vi "CMD_Loop.vi"() -> ()   [LabVIEW 2023, in "2023-Auto_CMD.lvlib"]
uses:
  2023-Auto_CMD.lvlib
  Cluster_CMD_CMD_Data.ctl
  Shared Code/TypeDefs/ENUM_AutoSelect.ctl
  ENUM_CMD_State.ctl
  ENUM_CMD_Action.ctl
  Shared Code/TypeDefs/Cluster_AutoSequence.ctl
  Shared Code/TypeDefs/Cluster_Auto Sequence Data.ctl
  Shared Code/TypeDefs/Cluster_Auto Sequence Settings.ctl
  ENUM_Drive Mode Select.ctl
  Shared Code/TypeDefs/Dial_Compase heading unit circle CCW positive.ctl
  Shared Code/TypeDefs/Cluster_Module Velocity-Direction-Rotations.ctl
  Shared Code/TypeDefs/Level_Velocity plus-minus 1.ctl
  SwerveDrive/Cluster_CMD_ACT_Data.ctl
  Shared Code/TypeDefs/ENUM_CMD_Mode Select.ctl
  Shared Code/TypeDefs/Cluster_CMD_Direction Data.ctl
  Shared Code/TypeDefs/Cluster_X-Y.ctl
  Shooter/Cluster_CMD_ACT_Data.ctl
  Shooter/ENUM_Shooter_Mode.ctl
  <vilib>/Rock Robotics/WPI/DriverStation/WPI_DriverStationRobotMode2.ctl
  Shared Code/TypeDefs/Cluster_Config_AutoData.ctl
  Pivot FX/Cluster_CMD_ACT_Data.ctl
  Pivot FX/ENUM_CMD_Mode Select.ctl
  Shared Code/TypeDefs/ENUM_Pivot Arm Position Select.ctl
  fdd46993-b9fc-440f-aafb-7ab1a8c35176.vi
  133b30be-2fcb-456e-b4b0-07f770c500ae.vi
  1ba0cf27-86ce-4142-8b65-bcb405614ff3.vi
  09229b25-3731-4416-b61c-801146eec302.vi
  c7d6c6c0-b27b-4b8b-8552-511dbe9cf3c3.vi
  dfaa9063-9cc7-40d1-a81d-c10c38088b54.vi
  fdd46993-b9fc-440f-aafb-7ab1a8c35176.vi/958b2683-dd4b-41b7-8ed1-41c95f63cef0.vi
  fdd46993-b9fc-440f-aafb-7ab1a8c35176.vi/95f5fa9b-6175-4b34-88ee-cece92c38279.vi
  133b30be-2fcb-456e-b4b0-07f770c500ae.vi/958b2683-dd4b-41b7-8ed1-41c95f63cef0.vi
  133b30be-2fcb-456e-b4b0-07f770c500ae.vi/95f5fa9b-6175-4b34-88ee-cece92c38279.vi
  09229b25-3731-4416-b61c-801146eec302.vi/958b2683-dd4b-41b7-8ed1-41c95f63cef0.vi
  09229b25-3731-4416-b61c-801146eec302.vi/95f5fa9b-6175-4b34-88ee-cece92c38279.vi
  c7d6c6c0-b27b-4b8b-8552-511dbe9cf3c3.vi/958b2683-dd4b-41b7-8ed1-41c95f63cef0.vi
  c7d6c6c0-b27b-4b8b-8552-511dbe9cf3c3.vi/95f5fa9b-6175-4b34-88ee-cece92c38279.vi
  <vilib>/Utility/error.llb/Trim Whitespace.vi
  fdd46993-b9fc-440f-aafb-7ab1a8c35176.vi/95f5fa9b-6175-4b34-88ee-cece92c38279.vi/1c6bd52c-bbca-4d4a-a290-93ea2703fded.vi
  fdd46993-b9fc-440f-aafb-7ab1a8c35176.vi/95f5fa9b-6175-4b34-88ee-cece92c38279.vi/47c2b0d5-b5fa-444e-9535-611565d375db.vi
  133b30be-2fcb-456e-b4b0-07f770c500ae.vi/95f5fa9b-6175-4b34-88ee-cece92c38279.vi/1c6bd52c-bbca-4d4a-a290-93ea2703fded.vi
  133b30be-2fcb-456e-b4b0-07f770c500ae.vi/95f5fa9b-6175-4b34-88ee-cece92c38279.vi/47c2b0d5-b5fa-444e-9535-611565d375db.vi
  09229b25-3731-4416-b61c-801146eec302.vi/95f5fa9b-6175-4b34-88ee-cece92c38279.vi/1c6bd52c-bbca-4d4a-a290-93ea2703fded.vi
  09229b25-3731-4416-b61c-801146eec302.vi/95f5fa9b-6175-4b34-88ee-cece92c38279.vi/47c2b0d5-b5fa-444e-9535-611565d375db.vi
  c7d6c6c0-b27b-4b8b-8552-511dbe9cf3c3.vi/95f5fa9b-6175-4b34-88ee-cece92c38279.vi/1c6bd52c-bbca-4d4a-a290-93ea2703fded.vi
  c7d6c6c0-b27b-4b8b-8552-511dbe9cf3c3.vi/95f5fa9b-6175-4b34-88ee-cece92c38279.vi/47c2b0d5-b5fa-444e-9535-611565d375db.vi
  <vilib>/Utility/error.llb/Trim Whitespace One-Sided.vi
  Robot Global Data.vi
  RoboRIO Utilities/Global_STOP.vi
  <vilib>/Utility/Data Type/Get Type Information.vi
  Shared Code/Utility/RWA/RWA/File/RWA_PC FIle Read String.vi
  Shared Code/Utility/RWA/RWA/Read Write Anything/RWA_File String.vi
  Shared Code/Utility/RWA/RWA/File/RWA_PC File Write String.vi
  Global_CMD_CMD_Data In.vi
  Shooter/Global_ACT_Data Out.vi
  SwerveDrive/Global_ACT_Data Out.vi
  Pivot FX/Global_ACT_Data Out.vi
  Pivot FX/Global_CMD_ACT_Data In.vi
  Shooter/Global_CMD_ACT_Data In.vi
  SwerveDrive/Global_CMD_ACT_Data In.vi
  Global_CMD_Data Out.vi
  <vilib>/Comparison/Equal/Equal Functor/Equal Functor.lvclass
  SwerveDrive/SwerveDrive_ACT_ts.lvlib
  Shooter/Shooter_ACT.lvlib
  Pivot FX/Pivot FX_ACT.lvlib
panel:
  out "Encoder .Position":i32
  out "Pivot at Position":bool
  out "Sequence Data":T1={"State"=enum."Starting", "Max Wait Time (S)"=0.0, "CMDs"={"Drive Mode"=enum."Wait", "Auto Angle"=0.0, "Traverse"={"Velocity"=0.0, "Angle"=0.0, "Rotations Count"=0.0}, "Shooter Speed"=0.0}, "Color Box"=16448250} {"CMDs"."Traverse"."Angle" scale format="%.3f"; "CMDs"."Traverse"."Velocity" scale=-1.0..1.0 scale format="%.1f"; "CMDs"."Auto Angle" scale format="%.3f"}
  out "CMD_Shooter":T8
  out "CMD_SwerveDrive":T10 {"Auto Angle" scale format="%.3f"; "Direction"."Rotate(Yaw) CCW 1 CW -1" scale=1.0..-1.0; "Direction"."Traverse"."Angle" scale format="%.3f"; "Direction"."Traverse"."Velocity" scale=-1.0..1.0 scale format="%.1f"}
  in  "AutoData.Sequences":T14[](array[typedef])=[{"Name"=enum."Unknown", "List"=[{"State"=enum."Driving to Position", "Max Wait Time (S)"=2.0, "CMDs"={"Drive Mode"=enum."Wait", "Auto Angle"=0.0, "Traverse"={"Velocity"=0.3, "Angle"=0.0, "Rotations Count"=0.0}, "Shooter Speed"=0.0}, "Color Box"=8404992}]}] {"List"."CMDs"."Traverse"."Angle" scale format="%.3f"; "List"."CMDs"."Traverse"."Velocity" scale=-1.0..1.0 scale format="%.1f"; "List"."CMDs"."Auto Angle" scale format="%.3f"}
  out "Remaing Match Time":sgl
  out "Step Index 2":i32
  out "CMD Input.Auto Select":T15=enum."Shoot and Drive Center"
  out "Found":bool
  out "Error Out":errorcluster
  out "Message Out":string
  in  "Read Saved Config":bool
  in  "Update Config":bool
  out "Action":T16
  out "State":T2
  out "Step Index":i32
  out "CMD_CMD_2022-Auto_Data":T17={"Auto Select"=enum."Shoot and Drive SpeakerLeft"}
  in  "Reset Sequence":bool
  in  "Reset All":bool
  in  "Set Manual":bool
  out "Input Data":T17={"Auto Select"=enum."Shoot and Drive SpeakerLeft"}
  out "Cycle Time (S)":dbl format="%.3g"
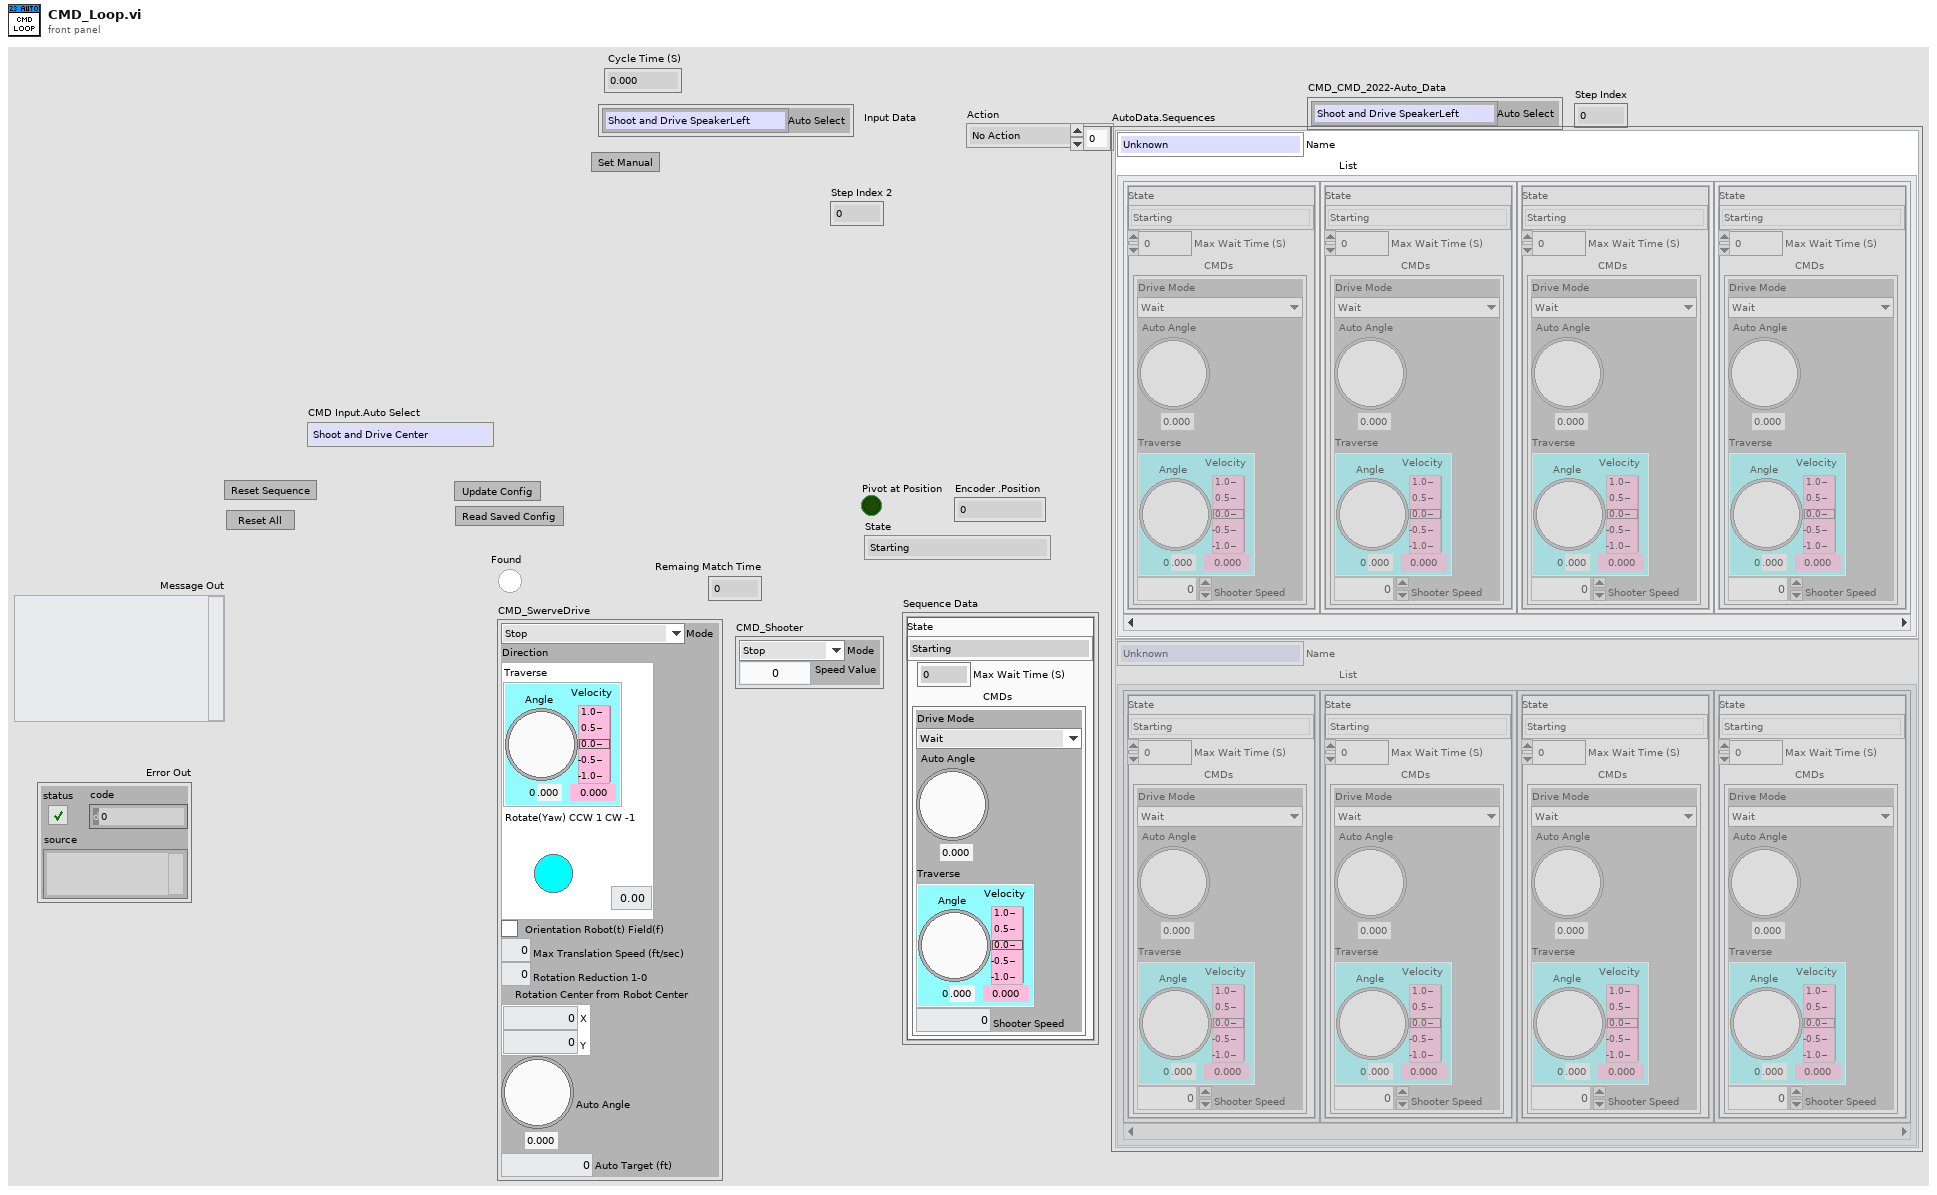
[diagram p1: front panel]
types:
  T1 = typedef "Cluster_Auto Sequence Data.ctl" = cluster{"State":T2, "Max Wait Time (S)":dbl, "CMDs":T3, "Color Box":u32}
  T2 = typedef "2023-Auto_CMD.lvlib/ENUM_CMD_State.ctl" = enum16{"Starting", "Idling", "Selecting Sequence", "Selecting Next Step", "Driving to Position", "Stopping", "Waiting", "Shutting Down", "Configuring", "Shooting", "Waiting for Pivot"}
  T3 = typedef "Cluster_Auto Sequence Settings.ctl" = cluster{"Drive Mode":T4, "Auto Angle":T5, "Traverse":T6, "Shooter Speed":dbl}
  T4 = typedef "2023-Auto_CMD.lvlib/ENUM_Drive Mode Select.ctl" = enum16{"Wait", "Timed Direction Drive", "Rotate to Angle", "Stop", "Auto Shoot"}
  T5 = typedef "Dial_Compase heading unit circle CCW positive.ctl" = dbl
  T6 = typedef "Cluster_Module Velocity-Direction-Rotations.ctl" = cluster{"Velocity":T7, "Angle":T5, "Rotations Count":dbl}
  T7 = typedef "Level_Velocity plus-minus 1.ctl" = dbl
  T8 = typedef "Shooter_ACT.lvlib/Cluster_CMD_ACT_Data.ctl" = cluster{"Mode":T9, "Speed Value":dbl}
  T9 = typedef "Shooter_ACT.lvlib/ENUM_Shooter_Mode.ctl" = enum16{"Stop", "Speed Percent", "Speed RPM", "AutoShoot"}
  T10 = typedef "SwerveDrive_ACT_ts.lvlib/Cluster_CMD_ACT_Data.ctl" = cluster{"Mode":T11, "Direction":T12, "Orientation Robot(t) Field(f)":bool, "Max Translation Speed (ft/sec)":dbl, "Rotation Reduction 1-0":dbl, "Rotation Center from Robot Center":T13, "Auto Angle":T5, "Auto Target (ft)":dbl}
  T11 = typedef "ENUM_CMD_Mode Select.ctl" = enum16{"Stop", "Translate Cmd Rotate Cmd", "Translate Cmd Rotate Auto"}
  T12 = typedef "Cluster_CMD_Direction Data.ctl" = cluster{"Traverse":T6, "Rotate(Yaw) CCW 1 CW -1":dbl}
  T13 = typedef "Cluster_X-Y.ctl" = cluster{"X":dbl, "Y":dbl}
  T14 = typedef "Cluster_AutoSequence.ctl" = cluster{"Name":T15, "List":T1[]}
  T15 = typedef "ENUM_AutoSelect.ctl" = enum16{"Unknown", "Shoot and Drive Center", "Shoot and Drive SpeakerLeft", "Shoot and Drive SpeakerRight"}
  T16 = typedef "2023-Auto_CMD.lvlib/ENUM_CMD_Action.ctl" = enum16{"No Action", "Reset Time", "Reset All", "Set System Cmds", "Reset Sequence", "Config File Read", "Config File Wirte", "Config from FP"}
  T17 = typedef "2023-Auto_CMD.lvlib/Cluster_CMD_CMD_Data.ctl" = cluster{"Auto Select":T15}
  T18 = typedef "Cluster_Config_AutoData.ctl" = cluster{"AutoData Ver":u64, "Sequences":T14[]}
  T19 = typedef "WPI_DriverStationRobotMode2.ctl" = enum16{"Autonomous Disabled", "Autonomous Enabled", "Teleop Disabled", "Teleop Enabled", "Disconnected", "Finish", "Test Disabled", "Test Enabled", "Emergency Stopped"}
  T20 = cluster{"State":T2, "Previous State":T2, "Current Time":timestamp, "Previous Time":timestamp, "Start Time":timestamp, "Target Time (ms)":u32, "Cycle Time(S)":dbl, "CMD Input":T17, "Sequence Array":T1[], "Step Data":T3, "Step Index":i32, "Robot Mode":T19, "Prev Robot Mode":T19, "Auto Select ":T15, "Team Files Folder":path, "AutoData":T18, "Update Display":bool, "Data Read":bool, "Remaing Match Time":sgl, "CMD_SwerveDrive":T10, "CMD_Shooter":T8, "AutoShootComplete":bool, "AutoAngleComplete":bool, "Pivot Out of the way":bool}
  T21 = typedef "Pivot FX_ACT.lvlib/Cluster_CMD_ACT_Data.ctl" = cluster{"Mode":T22, "Percent":dbl, "Target Position":dbl, "Position Select":T23}
  T22 = typedef "Pivot FX_ACT.lvlib/ENUM_CMD_Mode Select.ctl" = enum16{"STOP", "PercentOut", "Positon Value", "Position Select"}
  T23 = typedef "ENUM_Pivot Arm Position Select.ctl" = enum16{"Full Back", "Full Forward", "Amp Score", "Pivot Arm Load", "Vertical", "Trap Score"}
  T24 = typedef "SwerveDrive_ACT_ts.lvlib/Cluster_System Output Data.ctl" = cluster{"At Angle":bool}
  T25 = typedef "Pivot FX_ACT.lvlib/Cluster_HW Output Values.ctl" = cluster{"CLosed Loop":T26, "Current":T27, "Limit Switches":T28, "Voltage Values":T29, "Encoder ":T30}
  T26 = typedef "Cluster_FX CloseLoop Values.ctl" = cluster{"Target":dbl, "Error":i32, "Error D":dbl, "I Accum":dbl}
  T27 = typedef "Cluster_FX Current Values.ctl" = cluster{"Supply":dbl, "Stator":dbl}
  T28 = typedef "Cluster_FX Limit Switchs.ctl" = cluster{"FWD Closed":bool, "REV Closed":bool}
  T29 = typedef "Cluster_FX Voltage Values.ctl" = cluster{"Percent Output":dbl, "Output Voltage":dbl, "Bus Voltage":dbl}
  T30 = typedef "Cluster_FX Sensor Values.ctl" = cluster{"Position":i32, "Velocity":i32}
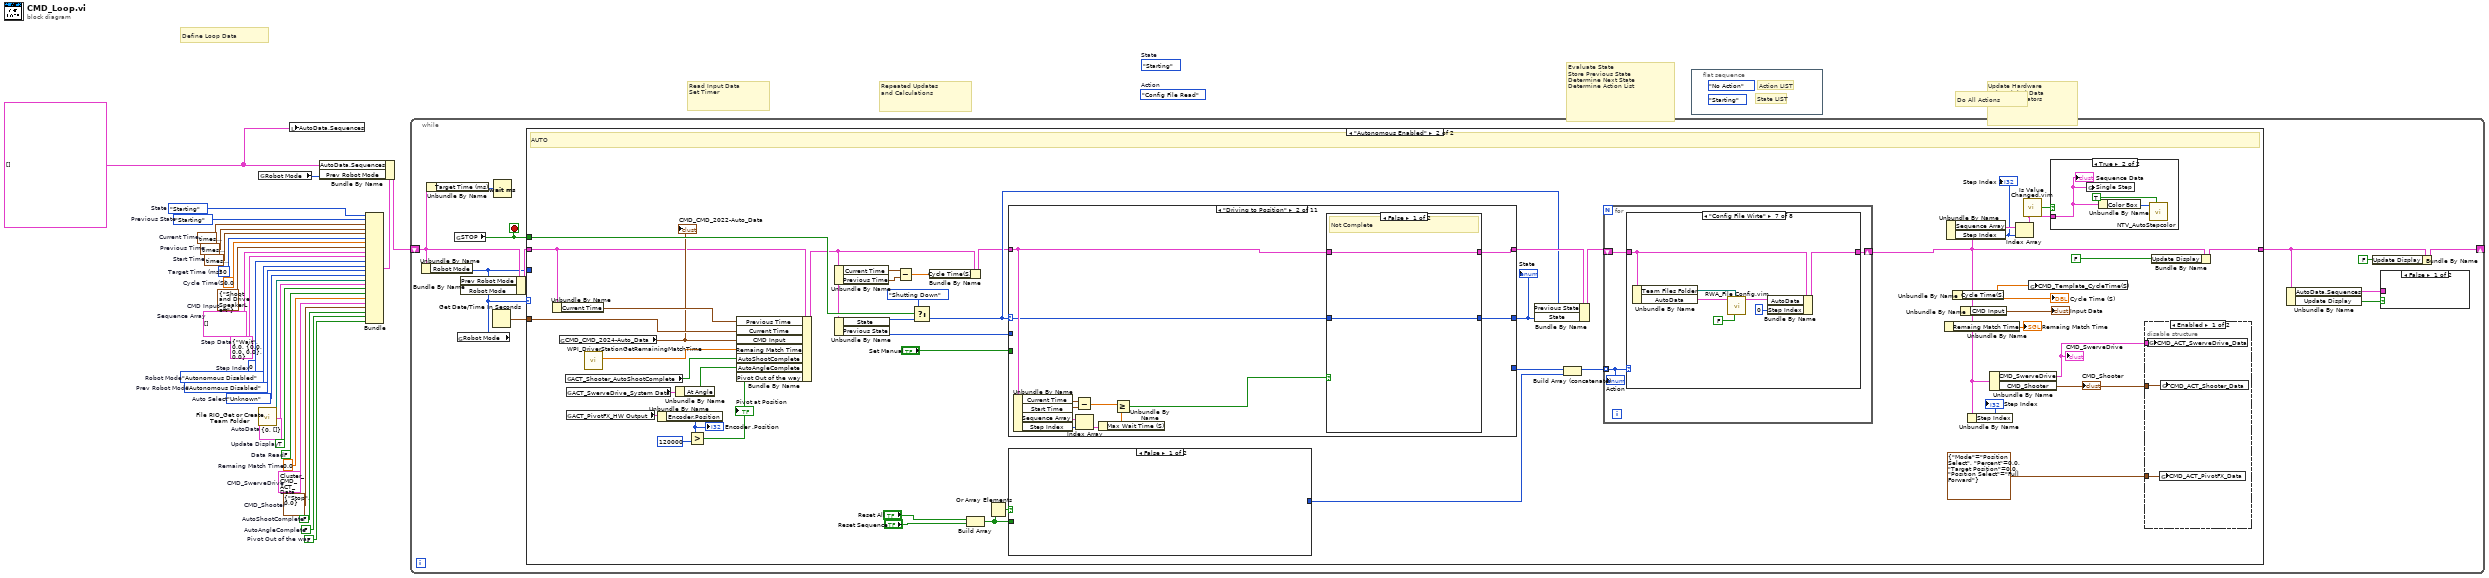
[diagram p0: block diagram]
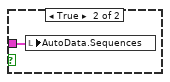
[diagram p2: hidden frame]
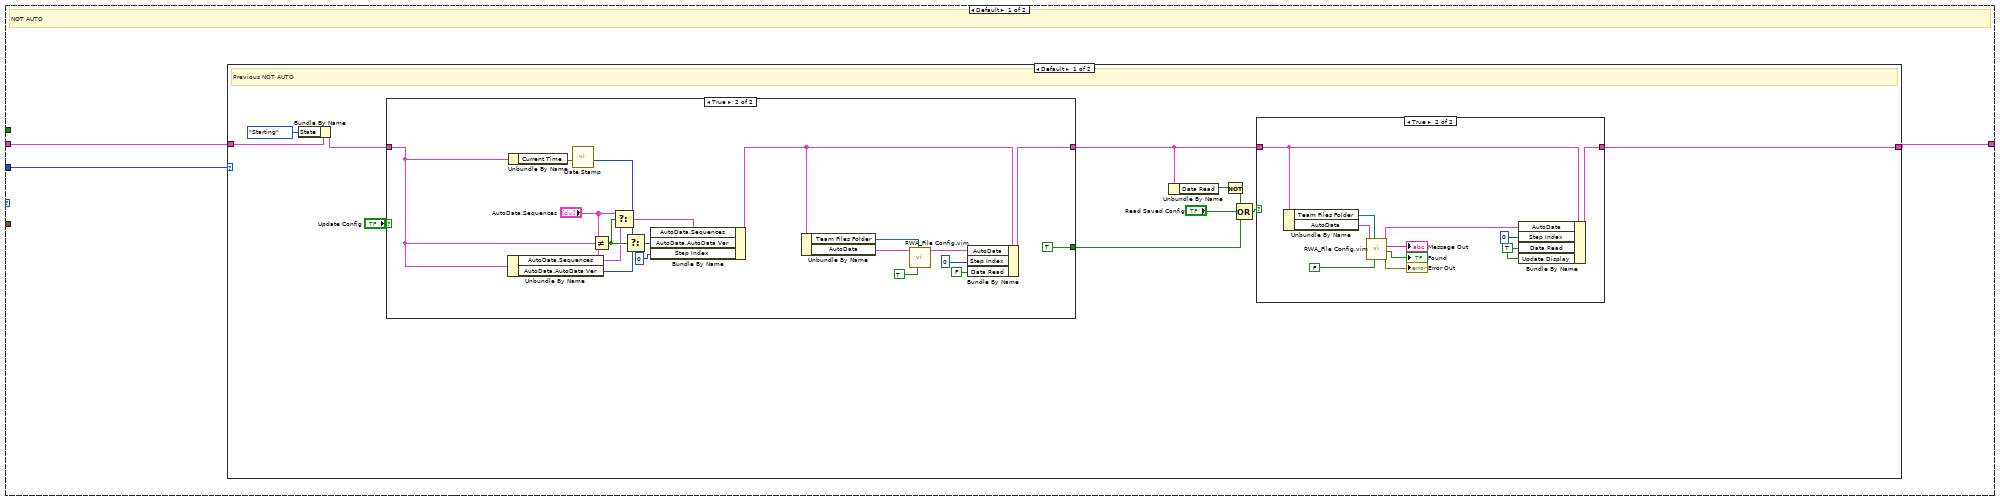
[diagram p3: hidden frame]
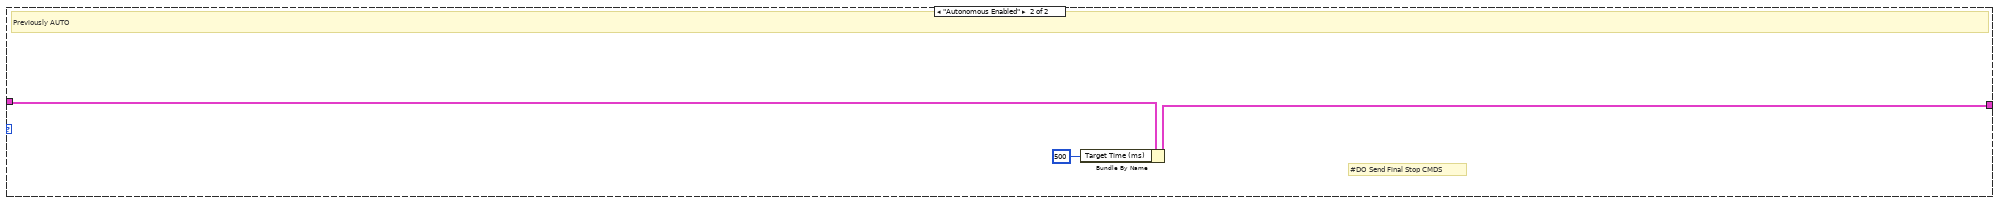
[diagram p6: hidden frame]
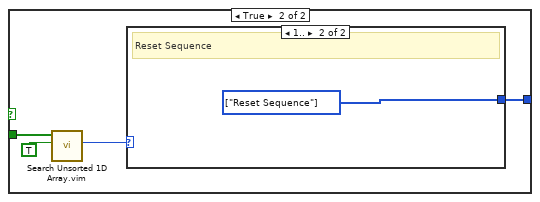
[diagram p8: hidden frame]
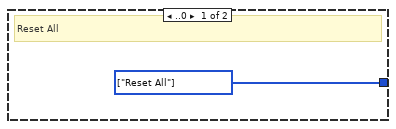
[diagram p9: hidden frame]
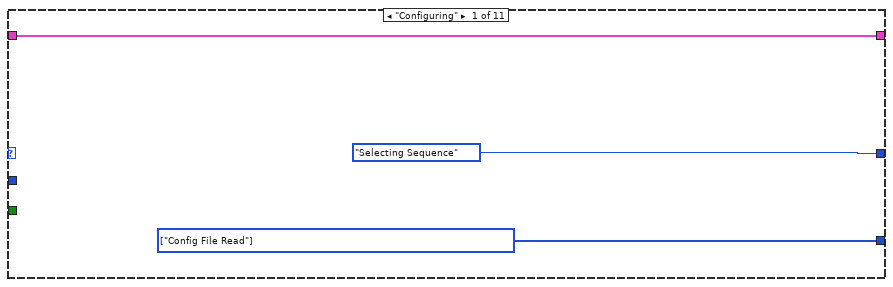
[diagram p10: hidden frame]
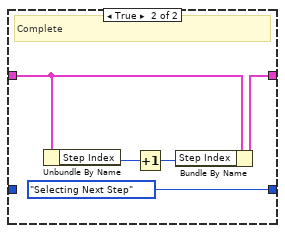
[diagram p11: hidden frame]
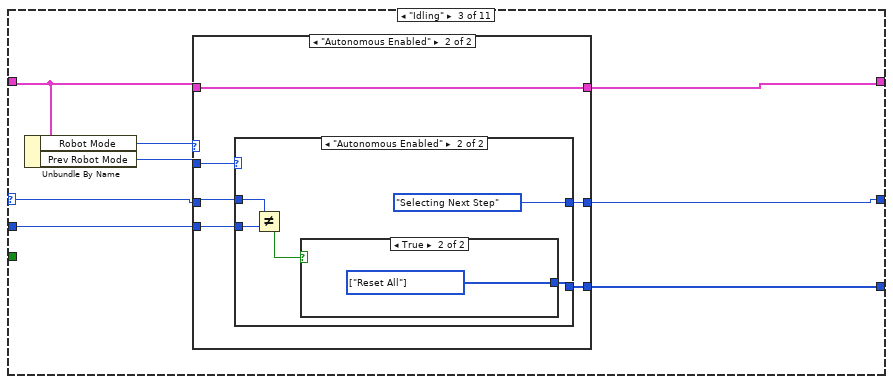
[diagram p12: hidden frame]
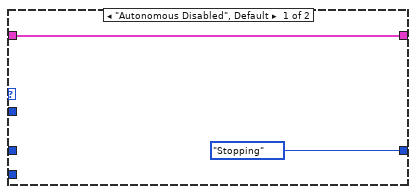
[diagram p13: hidden frame]
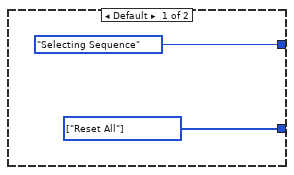
[diagram p14: hidden frame]
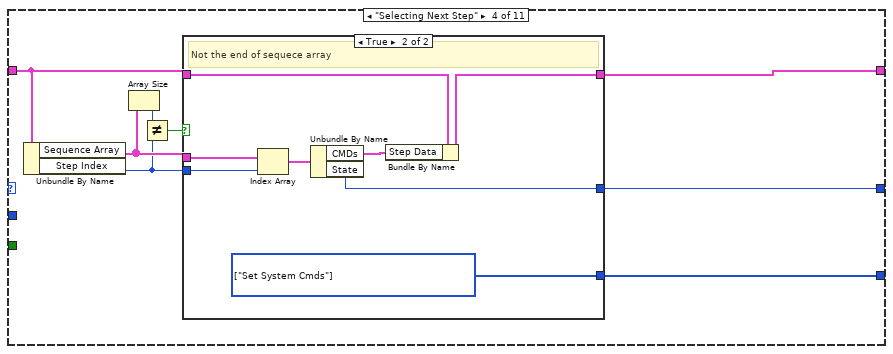
[diagram p16: hidden frame]
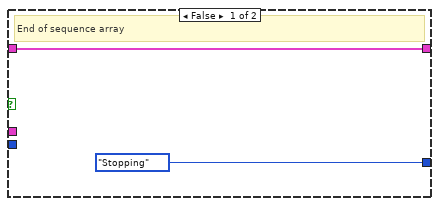
[diagram p17: hidden frame]
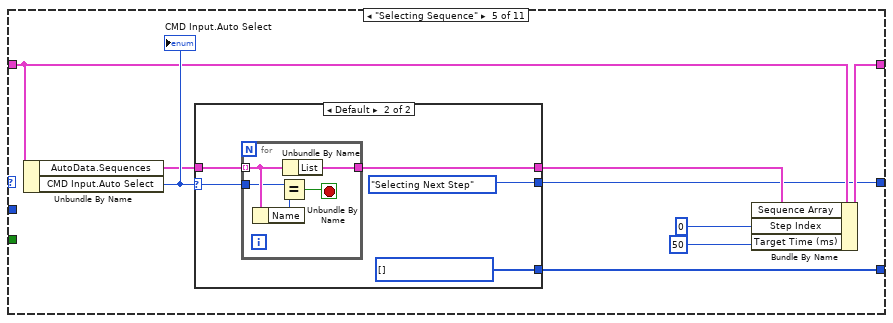
[diagram p18: hidden frame]
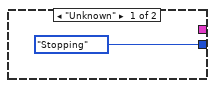
[diagram p19: hidden frame]
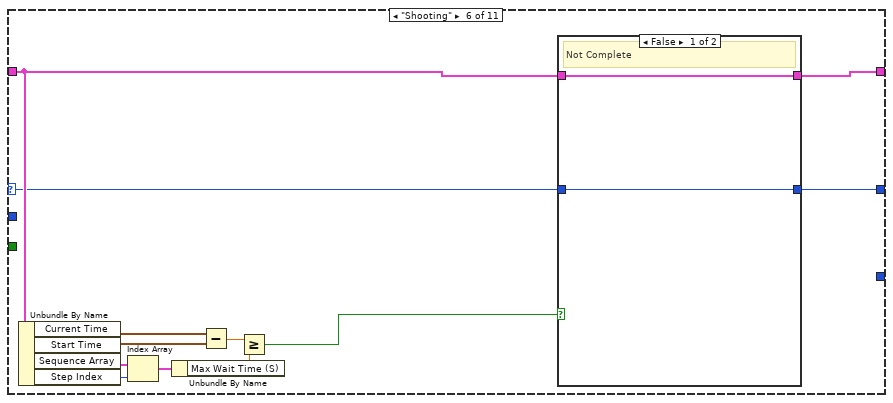
[diagram p20: hidden frame]
diagram:
  w1 = FALSE  # Pivot Out of the way
  w2 = FALSE  # AutoAngleComplete
  w3 = FALSE  # AutoShootComplete
  w4 = T8 {"Mode"=enum."Stop", "Speed Value"=0.0}  # CMD_Shooter
  w5 = T10 {"Mode"=enum."Stop", "Direction"={"Traverse"={"Velocity"=0.0, "Angle"=0.0, "Rotations Count"=0.0}, "Rotate(Yaw) CCW 1 CW -1"=0.0}, "Orientation Robot(t) Field(f)"=FALSE, "Max Translation Speed (ft/sec)"=0.0, "Rotation Reduction 1-0"=0.0, "Rotation Center from Robot Center"={"X"=0.0, "Y"=0.0}, "Auto Angle"=0.0, "Auto Target (ft)"=0.0}  # CMD_SwerveDrive
  w6 = T14[] [] ("AutoData.Sequences")
  (unwired) ENUM_CMD_State."Starting"  # State
  (unwired) ENUM_CMD_Action."Config File Read"  # Action
  w7 = sgl 0.0  # Remaing Match Time
  w8 = FALSE  # Data Read
  w9 = TRUE  # Update Display
  w10 = T18 {"AutoData Ver"=0, "Sequences"=[]}  # AutoData
  w12 = ENUM_AutoSelect."Unknown"  # Auto Select
  w16 = WPI_DriverStationRobotMode2."Autonomous Disabled"  # Prev Robot Mode
  w17 = WPI_DriverStationRobotMode2."Autonomous Disabled"  # Robot Mode
  w18 = 0  # Step Index
  w19 = T3 {"Drive Mode"=enum."Wait", "Auto Angle"=0.0, "Traverse"={"Velocity"=0.0, "Angle"=0.0, "Rotations Count"=0.0}, "Shooter Speed"=0.0}  # Step Data
  w20 = T1[] []  # Sequence Array
  w21 = 0.0  # Cycle Time(S)
  w22 = ENUM_CMD_State."Starting"  # Previous State
  w23 = timestamp(0 s since 1904-01-01)  # Previous Time
  w24 = u32 50  # Target Time (ms)
  w25 = T17 {"Auto Select"=enum."Shoot and Drive SpeakerLeft"}  # CMD Input
  w26 = timestamp(0 s since 1904-01-01)  # Start Time
  w27 = timestamp(0 s since 1904-01-01)  # Current Time
  w28 = ENUM_CMD_State."Starting"  # State
  # "Define Loop Data"
  # "Repeated Updates\nand Calculations"
  # "Read Input Data\nSet Timer"
  # "Evaluate State\nStore Previous State\nDetermine Next State\nDetermine Action List"
  # "Do All Actions"
  # "Update Hardware\nWrite Global Data\nUpdate Indicators"
  n1 = call "File RIO_Get or Create Team Folder.vi"() -> ("Team Files Folder"=w11:path)  [unwired: 10 in, 1 out]
  n2 = global read "Robot Global Data.vi" "Robot Mode"() -> (w13:T19)
  n3 = local write "AutoData.Sequences"(w6) -> ()
  n4 = Bundle("State"=w28, "Previous State"=w22, "Current Time"=w27, "Previous Time"=w23, "Start Time"=w26, "Target Time (ms)"=w24, "Cycle Time(S)"=w21, "CMD Input"=w25, "Sequence Array"=w20, "Step Data"=w19, "Step Index"=w18, "Robot Mode"=w17, "Prev Robot Mode"=w16, "Auto Select"=w12, "Team Files Folder"=w11, "AutoData"=w10, "Update Display"=w9, "Data Read"=w8, "Remaing Match Time"=w7, "CMD_SwerveDrive"=w5, "CMD_Shooter"=w4, "AutoShootComplete"=w3, "AutoAngleComplete"=w2, "Pivot Out of the way"=w1) -> (w15:T20)  [unwired: 1 in]
  n5 = Bundle By Name(cluster=w15, "AutoData.Sequences"=w6, "Prev Robot Mode"=w13) -> (w14:T20)
  n6 = while {
    shift-right: [w30] -> _
    shift-left: w14 -> [w37]
    stop <- w38 stop-if-true
    n7 = Unbundle By Name(w37) -> ("Robot Mode"=w35:T19)
    n8 = Unbundle By Name(w37) -> ("Target Time (ms)"=w39:u32)
    n9 = global read "Global_STOP.vi" "STOP"() -> (w38:bool)
    n10 = global read "Robot Global Data.vi" "Robot Mode"() -> (w34:T19)
    n11 = Bundle By Name(cluster=w37, "Prev Robot Mode"=w35, "Robot Mode"=w34) -> (w36:T20)
    n12 = Get Date/Time In Seconds() -> (seconds since 1Jan1904=w40:timestamp)
    n13 = Wait (ms)(milliseconds to wait=w39) -> ()  [unwired: 1 out]
    n14 = case shown="\"Autonomous Enabled\"" w34 {
      tunnel: w40 -> [_ w137]
      tunnel: [w43 w112] -> w31
      tunnel: w36 -> [w44 w105]
      tunnel: w35 -> [w42 _]
      tunnel: w38 -> [_ w119]
      frame Default {
        # "NOT AUTO"
        n15 = case shown="Default" w42 {
          tunnel: w44 -> [w55 w89]
          tunnel: [w49 w88] -> w43
          frame Default {
            # "Previous NOT AUTO"
            n16 = Bundle By Name(cluster=w55, "State"=ENUM_CMD_State."Starting") -> (w47:T20)
            n17 = case shown="True" "Update Config" {
              tunnel: w47 -> [w56 w67]
              tunnel: [w56 w59] -> w46
              tunnel: [_ TRUE] -> w45
              frame False {
              }
              frame True {
                n18 = Unbundle By Name(w67) -> ("AutoData.Sequences"=w70:T14[], "AutoData.AutoData Ver"=w73:u64)
                n19 = Unbundle By Name(w67) -> ("Current Time"=w75:timestamp)
                n20 = call "Date Stamp.vi"("Time"=w75) -> ("U64 Out"=w74:u64)  [unwired: 5 in, 1 out]
                n21 = Not Equal?(x="AutoData.Sequences", y=w70) -> (x != y?=w71:bool)
                n22 = Select(t="AutoData.Sequences", s=w71, f=w70) -> (s? t:f=w69:T14[])
                n23 = Select(t=w74, s=w71, f=w73) -> (s? t:f=w72:u64)
                n24 = Bundle By Name(cluster=w67, "AutoData.Sequences"=w69, "AutoData.AutoData Ver"=w72, "Step Index"=0) -> (w60:T20)
                n25 = Unbundle By Name(w60) -> ("Team Files Folder"=w65:path, "AutoData"=w64:T18)
                n26 = call "RWA_File Config.vim"("Read(f) Save(t)"=TRUE ("Read(f) Write(t)"), "Target Folder Folder"=w65, "Any Config"=w64) -> ("Any Config Out"=w66:T18)  [unwired: 4 in, 4 out]
                n27 = Bundle By Name(cluster=w60, "AutoData"=w66, "Step Index"=0, "Data Read"=FALSE) -> (w59:T20)
              }
            }
            n28 = Unbundle By Name(w46) -> ("Data Read"=w53:bool)
            n29 = Not(x=w53) -> (.not. x?=w52:bool)
            n30 = Compound Arithmetic op=OR(w52, "Read Saved Config", w45) -> (w50:bool)
            n31 = case shown="True" w50 {
              tunnel: w46 -> [w76 w86]
              tunnel: [w76 w85] -> w49
              frame False {
              }
              frame True {
                w84 = TRUE ("Data Read")
                n32 = Unbundle By Name(w86) -> ("Team Files Folder"=w79:path, "AutoData"=w83:T18)
                n33 = call "RWA_File Config.vim"("Read(f) Save(t)"=FALSE ("Read(f) Write(t)"), "Target Folder Folder"=w79, "Any Config"=w83) -> ("Error Out"=→"Error Out":errorcluster, "Found Out"=→"Found":bool, "Message Out"=→"Message Out":string, "Any Config Out"=w82:T18)  [unwired: 4 in, 1 out]
                n34 = Bundle By Name(cluster=w86, "AutoData"=w82, "Step Index"=0, "Data Read"=w84, "Update Display"=w84) -> (w85:T20)
              }
            }
          }
          frame "Autonomous Enabled" {
            # "#DO Send Final Stop CMDS"
            # "Previously AUTO"
            n35 = Bundle By Name(cluster=w89, "Target Time (ms)"=u32 500) -> (w88:T20)
          }
        }
      }
      frame "Autonomous Enabled" {
        # "AUTO"
        n36 = Unbundle By Name(w105) -> ("Current Time"=w113:timestamp)
        n37 = global read "Global_CMD_CMD_Data In.vi" "CMD_CMD_2024-Auto_Data"() -> (w106:T17)
        "CMD_CMD_2022-Auto_Data" <- w106
        n38 = global read "Global_ACT_Data Out.vi" "ACT_Shooter_AutoShootComplete"() -> (w98:bool)
        n39 = global read "Global_ACT_Data Out.vi" "ACT_SwerveDrive_System Data"() -> (w97:T24)
        n40 = global read "Global_ACT_Data Out.vi" "ACT_PivotFX_HW Output"() -> (w95:T25)
        n41 = call <vilib>:"WPI_DriverStationGetRemainingMatchTime.vi"() -> ("Match Time(s)"=w104:sgl)  [unwired: 10 in, 1 out]
        n42 = Unbundle By Name(w95) -> ("Encoder.Position"=w93:i32)
        "Encoder .Position" <- w93
        n43 = Unbundle By Name(w97) -> ("At Angle"=w96:bool)
        n44 = Greater?(x=w93, y=120000) -> (0:w91:bool)
        "Pivot at Position" <- w91
        n45 = Bundle By Name(cluster=w105, "Previous Time"=w113, "Current Time"=w137, "CMD Input"=w106, "Remaing Match Time"=w104, "AutoShootComplete"=w98, "AutoAngleComplete"=w96, "Pivot Out of the way"=w91) -> (w102:T20)
        n46 = Unbundle By Name(w102) -> ("State"=w132:T2, "Previous State"=w131:T2)
        n47 = Unbundle By Name(w102) -> ("Current Time"=w128:timestamp, "Previous Time"=w129:timestamp)
        n48 = Subtract(x=w128, y=w129) -> (x-y=w126:dbl)
        n49 = Select(t=ENUM_CMD_State."Shutting Down" ("State"), s=w119, f=w132) -> (s? t:f=w130:T2)
        n50 = Bundle By Name(cluster=w102, "Cycle Time(S)"=w126) -> (w127:T20)
        n51 = Build Array("Reset All", "Reset Sequence") -> (w107:bool[])
        n52 = Or Array Elements(Boolean array=w107) -> (logical OR=w108:bool)
        n53 = case shown="\"Driving to Position\"" w130 {
          selector: w130 -> [_ w151 w174 _ _ w232 w257 _ _ _ w285]
          tunnel: w127 -> [w149 w152 w170 w197 w217 w235 w255 w276 w278 w282 w288]
          tunnel: [w149 w155 w169 w200 w218 w234 w259 w276 w279 w282 w287] -> w135
          tunnel: [ENUM_CMD_State."Selecting Sequence" ("State") w154 w172 w199 w214 w233 w258 ENUM_CMD_State."Shutting Down" ("State") ENUM_CMD_State."Selecting Sequence" ("State") ENUM_CMD_State."Idling" ("State") w286] -> w134
          tunnel: [w147 _ w176 w198 w213 _ _ w274 w281 _ _] -> w125
          tunnel: w131 -> [_ _ w175 _ _ _ _ _ _ _ _]
          tunnel: "Set Manual" -> [_ _ _ _ _ _ _ _ _ _ _]
          frame "Configuring" {
            w147 = T16[] [enum."Config File Read"] items=["No Action", "Reset Time", "Reset All", "Set System Cmds", "Reset Sequence", "Config File Read", "Config File Wirte", "Config from FP"] ("Actions")
          }
          frame "Driving to Position" {
            n54 = Unbundle By Name(w152) -> ("Current Time"=w158:timestamp, "Start Time"=w157:timestamp, "Sequence Array"=w161:T1[], "Step Index"=w160:i32)
            n55 = Subtract(x=w158, y=w157) -> (x-y=w156:dbl)
            n56 = Index Array(array=w161, index=w160) -> (element=w159:T1)
            n57 = Unbundle By Name(w159) -> ("Max Wait Time (S)"=w153:dbl)
            n58 = Greater Or Equal?(x=w156, y=w153) -> (x >= y?=w150:bool)
            n59 = case shown="False" w150 {
              tunnel: [w163 w166] -> w155
              tunnel: w152 -> [w163 w167]
              tunnel: [w162 ENUM_CMD_State."Selecting Next Step" ("State")] -> w154
              tunnel: w151 -> [w162 _]
              frame False {
                # "Not Complete"
              }
              frame True {
                # "Complete"
                n60 = Unbundle By Name(w167) -> ("Step Index"=w165:i32)
                n61 = Increment(x=w165) -> (x+1=w164:i32)
                n62 = Bundle By Name(cluster=w167, "Step Index"=w164) -> (w166:T20)
              }
            }
          }
          frame "Idling" {
            n63 = Unbundle By Name(w170) -> ("Robot Mode"=w173:T19, "Prev Robot Mode"=w171:T19)
            n64 = case shown="\"Autonomous Enabled\"" w173 {
              tunnel: [_ w184] -> w176
              tunnel: w175 -> [_ w183]
              tunnel: w174 -> [_ w182]
              tunnel: [ENUM_CMD_State."Stopping" ("State") w180] -> w172
              tunnel: w171 -> [_ w181]
              tunnel: w170 -> [w177 w179]
              tunnel: [w177 w179] -> w169
              frame "Autonomous Disabled", Default {
              }
              frame "Autonomous Enabled" {
                n65 = case shown="\"Autonomous Enabled\"" w181 {
                  tunnel: [w185 w191] -> w184
                  tunnel: w183 -> [_ w190]
                  tunnel: w182 -> [_ w189]
                  tunnel: [ENUM_CMD_State."Selecting Sequence" ("State") ENUM_CMD_State."Selecting Next Step" ("State")] -> w180
                  frame Default {
                    w185 = T16[] [enum."Reset All"] items=["No Action", "Reset Time", "Reset All", "Set System Cmds", "Reset Sequence", "Config File Read", "Config File Wirte", "Config from FP"] ("Actions")
                  }
                  frame "Autonomous Enabled" {
                    n66 = Not Equal?(x=w189, y=w190) -> (x != y?=w188:bool)
                    n67 = case shown="True" w188 {
                      tunnel: [_ w192] -> w191
                      frame False {
                      }
                      frame True {
                        w192 = T16[] [enum."Reset All"] items=["No Action", "Reset Time", "Reset All", "Set System Cmds", "Reset Sequence", "Config File Read", "Config File Wirte", "Config from FP"] ("Actions")
                      }
                    }
                  }
                }
              }
            }
          }
          frame "Selecting Next Step" {
            n68 = Unbundle By Name(w197) -> ("Sequence Array"=w196:T1[], "Step Index"=w195:i32)
            n69 = Array Size(array=w196) -> (size(s)=w194:i32)
            n70 = Not Equal?(x=w194, y=w195) -> (x != y?=w193:bool)
            n71 = case shown="True" w193 {
              tunnel: [w202 w210] -> w200
              tunnel: w197 -> [w202 w208]
              tunnel: [ENUM_CMD_State."Stopping" ("State") w206] -> w199
              tunnel: [_ w205] -> w198
              tunnel: w196 -> [_ w204]
              tunnel: w195 -> [_ w203]
              frame False {
                # "End of sequence array"
              }
              frame True {
                w205 = T16[] [enum."Set System Cmds"] items=["No Action", "Reset Time", "Reset All", "Set System Cmds", "Reset Sequence", "Config File Read", "Config File Wirte", "Config from FP"] ("Actions")
                # "Not the end of sequece array"
                n72 = Index Array(array=w204, index=w203) -> (element=w209:T1)
                n73 = Unbundle By Name(w209) -> ("CMDs"=w207:T3, "State"=w206:T2)
                n74 = Bundle By Name(cluster=w208, "Step Data"=w207) -> (w210:T20)
              }
            }
          }
          frame "Selecting Sequence" {
            n75 = Unbundle By Name(w217) -> ("AutoData.Sequences"=w211:T14[], "CMD Input.Auto Select"=w219:T15)
            "CMD Input.Auto Select" <- w219
            n76 = case shown="Default" w219 {
              selector: w219 -> [_ w222]
              tunnel: [_ w223] -> w216
              tunnel: [ENUM_CMD_State."Stopping" ("State") ENUM_CMD_State."Selecting Next Step" ("State")] -> w214
              tunnel: [_ w221] -> w213
              tunnel: w211 -> [_ w224]
              frame "Unknown" {
              }
              frame Default {
                w221 = T16[] [] items=["No Action", "Reset Time", "Reset All", "Set System Cmds", "Reset Sequence", "Config File Read", "Config File Wirte", "Config from FP"] ("Actions")
                n77 = for {
                  tunnel: w224 -> [w230] mode=indexing
                  tunnel: w222 -> [w228]
                  tunnel: [w229] -> w223
                  stop <- w226 stop-if-true
                  n78 = Unbundle By Name(w230) -> ("Name"=w227:T15)
                  n79 = Equal?(x=w228, y=w227) -> (x = y?=w226:bool)
                  n80 = Unbundle By Name(w230) -> ("List"=w229:T1[])
                }
              }
            }
            n81 = Bundle By Name(cluster=w217, "Sequence Array"=w216, "Step Index"=0, "Target Time (ms)"=u32 50) -> (w218:T20)
          }
          frame "Shooting" {
            n82 = Unbundle By Name(w235) -> ("Current Time"=w239:timestamp, "Start Time"=w238:timestamp, "Sequence Array"=w242:T1[], "Step Index"=w241:i32)
            n83 = Index Array(array=w242, index=w241) -> (element=w240:T1)
            n84 = Unbundle By Name(w240) -> ("Max Wait Time (S)"=w236:dbl)
            n85 = Subtract(x=w239, y=w238) -> (x-y=w237:dbl)
            n86 = Greater Or Equal?(x=w237, y=w236) -> (x >= y?=w231:bool)
            n87 = case shown="False" w231 {
              tunnel: [w244 w247] -> w234
              tunnel: w235 -> [w244 w248]
              tunnel: [w243 ENUM_CMD_State."Selecting Next Step" ("State")] -> w233
              tunnel: w232 -> [w243 _]
              frame False {
                # "Not Complete"
              }
              frame True {
                # "Complete"
                n88 = Unbundle By Name(w248) -> ("Step Index"=w246:i32)
                n89 = Increment(x=w246) -> (x+1=w245:i32)
                n90 = Bundle By Name(cluster=w248, "Step Index"=w245) -> (w247:T20)
              }
            }
          }
          frame "Waiting for Pivot" {
            n91 = Unbundle By Name(w255) -> ("Current Time"=w263:timestamp, "Start Time"=w262:timestamp, "Sequence Array"=w266:T1[], "Step Index"=w265:i32)
            n92 = Unbundle By Name(w255) -> ("Pivot Out of the way"=w254:bool)
            n93 = Index Array(array=w266, index=w265) -> (element=w264:T1)
            n94 = Unbundle By Name(w264) -> ("Max Wait Time (S)"=w260:dbl)
            n95 = Subtract(x=w263, y=w262) -> (x-y=w261:dbl)
            n96 = call "Bool_Delay OnOFF.vi"("Delay Time(S)"=0.1, "Delay On(t) Off(f)"=TRUE, "Input"=w254) -> ("Output"=w250:bool)  [unwired: 7 in, 1 out]
            n97 = Greater Or Equal?(x=w261, y=w260) -> (x >= y?=w256:bool)
            n98 = Or(x=w250, y=w256) -> (x .or. y?=w251:bool)
            n99 = case shown="False" w251 {
              tunnel: [w268 w271] -> w259
              tunnel: w255 -> [w268 w272]
              tunnel: [w267 ENUM_CMD_State."Selecting Next Step" ("State")] -> w258
              tunnel: w257 -> [w267 _]
              frame False {
                # "Not Complete"
              }
              frame True {
                # "Complete"
                n100 = Unbundle By Name(w272) -> ("Step Index"=w270:i32)
                n101 = Increment(x=w270) -> (x+1=w269:i32)
                n102 = Bundle By Name(cluster=w272, "Step Index"=w269) -> (w271:T20)
              }
            }
          }
          frame "Shutting Down" {
            w274 = T16[] [enum."Reset All"] items=["No Action", "Reset Time", "Reset All", "Set System Cmds", "Reset Sequence", "Config File Read", "Config File Wirte", "Config from FP"] ("Actions")
          }
          frame "Starting" {
            w281 = T16[] [enum."Reset Time"] items=["No Action", "Reset Time", "Reset All", "Set System Cmds", "Reset Sequence", "Config File Read", "Config File Wirte", "Config from FP"] ("Actions")
            n103 = Bundle By Name(cluster=w278, "Target Time (ms)"=u32 50) -> (w279:T20)
          }
          frame "Stopping" {
          }
          frame "Waiting" {
            n104 = Unbundle By Name(w288) -> ("Current Time"=w292:timestamp, "Start Time"=w291:timestamp, "Sequence Array"=w295:T1[], "Step Index"=w294:i32)
            n105 = Index Array(array=w295, index=w294) -> (element=w293:T1)
            n106 = Unbundle By Name(w293) -> ("Max Wait Time (S)"=w289:dbl)
            n107 = Subtract(x=w292, y=w291) -> (x-y=w290:dbl)
            n108 = Greater Or Equal?(x=w290, y=w289) -> (x >= y?=w284:bool)
            n109 = case shown="False" w284 {
              tunnel: [w297 w300] -> w287
              tunnel: w288 -> [w297 w301]
              tunnel: [w296 ENUM_CMD_State."Selecting Next Step" ("State")] -> w286
              tunnel: w285 -> [w296 _]
              frame False {
                # "Not Complete"
              }
              frame True {
                # "Complete"
                n110 = Unbundle By Name(w301) -> ("Step Index"=w299:i32)
                n111 = Increment(x=w299) -> (x+1=w298:i32)
                n112 = Bundle By Name(cluster=w301, "Step Index"=w298) -> (w300:T20)
              }
            }
          }
        }
        "State" <- w134
        n113 = case shown="False" w108 {
          tunnel: [_ w144] -> w121
          tunnel: w107 -> [_ w143]
          frame False {
          }
          frame True {
            n114 = call "Search Unsorted 1D Array.vim"("element"=TRUE, "unsorted 1D array"=w143) -> ("index of element"=w141:i32)  [unwired: 9 in]
            n115 = case shown="1.." w141 {
              tunnel: [w145 w146] -> w144
              frame ..0 {
                w145 = T16[] [enum."Reset All"] items=["No Action", "Reset Time", "Reset All", "Set System Cmds", "Reset Sequence", "Config File Read", "Config File Wirte", "Config from FP"] ("Actions")
                # "Reset All"
              }
              frame 1.. {
                w146 = T16[] [enum."Reset Sequence"] items=["No Action", "Reset Time", "Reset All", "Set System Cmds", "Reset Sequence", "Config File Read", "Config File Wirte", "Config from FP"] ("Actions")
                # "Reset Sequence"
              }
            }
          }
        }
        n116 = Bundle By Name(cluster=w135, "Previous State"=w130, "State"=w134) -> (w136:T20)
        n117 = Build Array (concatenate)(w125, w121) -> (w122:T16[])
        n118 = for {
          tunnel: w122 -> [w305] mode=indexing
          shift-right: [w304] -> w101
          shift-left: w136 -> [w303]
          n119 = case shown="\"Config File Wirte\"" w305 {
            tunnel: w303 -> [w306 w309 w314 w316 w317 w319 w324 w330]
            tunnel: [w306 w308 w315 w316 w317 w320 w325 w331] -> w304
            frame "No Action" {
            }
            frame "Reset Time" {
              # "Reset timer by taking the current time\nand making it the start time\n\nLater when the current time is \nsubtracted from the start time\nyou will get the elapsed time in \nseconds"
              n120 = Unbundle By Name(w309) -> ("Current Time"=w307:timestamp)
              n121 = Bundle By Name(cluster=w309, "Start Time"=w307) -> (w308:T20)
            }
            frame "Set System Cmds" {
              n122 = Unbundle By Name(w314) -> ("Current Time"=w312:timestamp, "Step Data"=w313:T3)
              n123 = call "Sequence Data to Sytem CMDs.vi"("Sequence Data"=w313) -> ("CMD_ACT_Drive_Data Out"=w310:T10, "CMD_ACT_shooter_Data"=w311:T8)  [unwired: 8 in, 1 out]
              n124 = Bundle By Name(cluster=w314, "Start Time"=w312, "CMD_Shooter"=w311, "CMD_SwerveDrive"=w310) -> (w315:T20)
            }
            frame "Config File Read" {
            }
            frame "Reset All" {
            }
            frame "Reset Sequence" {
              n125 = Bundle By Name(cluster=w319, "State"=ENUM_CMD_State."Selecting Sequence") -> (w320:T20)
            }
            frame "Config File Wirte" {
              n126 = Unbundle By Name(w324) -> ("Team Files Folder"=w326:path, "AutoData"=w327:T18)
              n127 = call "RWA_File Config.vim"("Read(f) Save(t)"=FALSE ("Read(f) Write(t)"), "Target Folder Folder"=w326, "Any Config"=w327) -> ("Any Config Out"=w323:T18)  [unwired: 4 in, 4 out]
              n128 = Bundle By Name(cluster=w324, "AutoData"=w323, "Step Index"=0) -> (w325:T20)
            }
            frame "Config from FP" {
              n129 = Unbundle By Name(w330) -> ("Team Files Folder"=w332:path, "AutoData"=w333:T18)
              n130 = call "RWA_File Config.vim"("Read(f) Save(t)"=TRUE ("Read(f) Write(t)"), "Target Folder Folder"=w332, "Any Config"=w333) -> ("Any Config Out"=w329:T18)  [unwired: 4 in, 4 out]
              n131 = Bundle By Name(cluster=w330, "AutoData"=w329) -> (w331:T20)
            }
          }
          "Action" <- w305
        }
        n132 = Unbundle By Name(w101) -> ("Remaing Match Time"=→"Remaing Match Time":sgl)
        n133 = Unbundle By Name(w101) -> ("Sequence Array"=w118:T1[], "Step Index"=w117:i32)
        "Step Index 2" <- w117
        n134 = Unbundle By Name(w101) -> ("Cycle Time(S)"=w123:dbl)
        "Cycle Time (S)" <- w123
        n135 = Unbundle By Name(w101) -> ("CMD Input"=→"Input Data":T17)
        n136 = Unbundle By Name(w101) -> ("Step Index"=→"Step Index":i32)
        n137 = Unbundle By Name(w101) -> ("CMD_SwerveDrive"=w100:T10, "CMD_Shooter"=w99:T8)
        "CMD_SwerveDrive" <- w100
        "CMD_Shooter" <- w99
        n138 = Index Array(array=w118, index=w117) -> (element=w115:T1)
        n139 = call "Is Value Changed.vim"("value"=w115) -> ("changed or first call?"=w116:bool)
        n140 = global write "Global_CMD_Data Out.vi" "CMD_Template_CycleTime(S)"(w123) -> ()
        n141 = case shown="True" w116 {
          tunnel: w115 -> [_ w336]
          frame False {
          }
          frame True {
            n142 = global write "Global_CMD_Data Out.vi" "Single Step"(w336) -> ()
            n143 = Unbundle By Name(w336) -> ("Color Box"=w334:u32)
            n144 = call "NTV_AutoStepcolor.vi"("Read(f) Write(t)"=TRUE, "Color"=w334) -> ()  [unwired: 9 in, 1 out]
            "Sequence Data" <- w336
          }
        }
        n145 = disable-structure shown="Enabled" {
          disable-tunnel: w100 -> [w140 _]
          disable-tunnel: w99 -> [w139 _]
          disable-tunnel: T21 {"Mode"=enum."Position Select", "Percent"=0.0, "Target Position"=0.0, "Position Select"=enum."Full Forward"} ("CMD_ACT_PivotFX_Data") -> [w138 _]
          frame Enabled {
            n146 = global write "Global_CMD_ACT_Data In.vi" "CMD_ACT_SwerveDrive_Data"(w140) -> ()
            n147 = global write "Global_CMD_ACT_Data In.vi" "CMD_ACT_PivotFX_Data"(w138) -> ()
            n148 = global write "Global_CMD_ACT_Data In.vi" "CMD_ACT_Shooter_Data"(w139) -> ()
          }
          frame Disabled {
          }
        }
        n149 = Bundle By Name(cluster=w101, "Update Display"=FALSE) -> (w112:T20)
      }
    }
    n150 = Unbundle By Name(w31) -> ("AutoData.Sequences"=w33:T14[], "Update Display"=w32:bool)
    n151 = Bundle By Name(cluster=w31, "Update Display"=FALSE) -> (w30:T20)
    n152 = case shown="False" w32 {
      tunnel: w33 -> [_ w41]
      frame False {
      }
      frame True {
        n153 = local write "AutoData.Sequences"(w41) -> ()
      }
    }
  }
  n154 = flat-sequence {
    frame #0 {
      (unwired) ENUM_CMD_State."Starting" ("State")
      (unwired) ENUM_CMD_Action."No Action" ("Action")
      # "State LIST"
      # "Action LIST"
    }
  }
